vi "CALC_DATA.vi"(0 "VISA IN":refnum<visa-resource-name>="GPIB1::16::INSTR", 5 "error in":errorcluster, 7 "Channel":i32=1, 11 "DataType":string="FDATA") -> (14 "VISA Out":refnum<visa-resource-name>="GPIB1::16::INSTR", 16 "array":dbl[](array[numeric]), 19 "error out":errorcluster={"status"=TRUE, "code"=-1073807339, "source"="VISA Read in CALC_DATA.vi"})   [LabVIEW 2018, in "PNA-X.lvlib"]
doc: "CALCulate<cnum>:DATA:CUSTom <name>,<data> \n(Read-Write) Reads or writes data from a custom-named measurement buffer. \nSee Critical Note \nParameters \n<cnum> Channel number of the measurement. There must be a selected measurement \non that channel. If unspecified, <cnum> is set to 1. \n<name> Name of the buffer to be read or written \n<data> Data to be read or written to the custom buffer. Format as one number per data \npoint. \nExamples CALC:DATA:CUST 'VectorResult0',0,1,2,3,4,5 'Write \nCALC:DATA:CUST? 'VectorResult0' 'Read \nQuery Syntax CALCulate:DATA:CUSTom? <name> \nReturn Type Depends on Form:Data \nDefault Not Applicable"
uses:
  PNA-X.lvlib
panel:
  out "Waveform Chart":dbl[](graph)
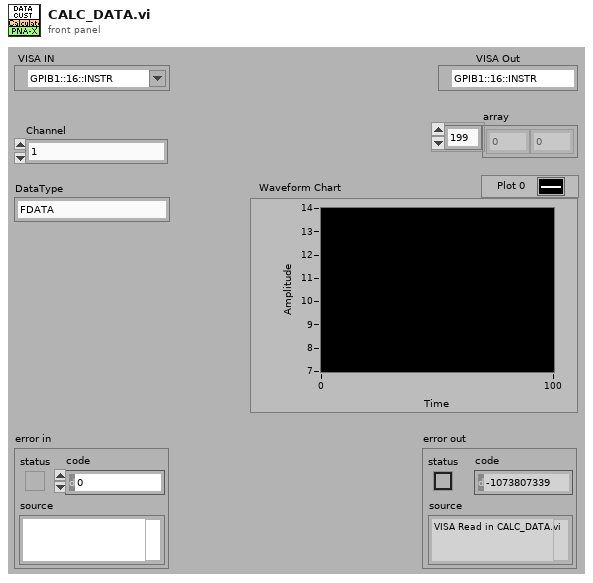
[diagram p1: front panel]
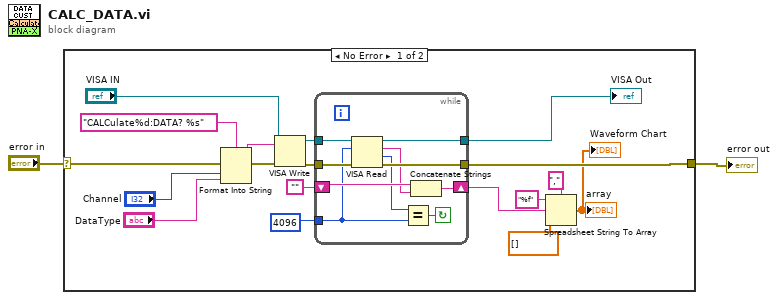
[diagram p0: block diagram]
diagram:
  n1 = case shown="No Error" "error in" {
    selector: "error in" -> [w20 w31]
    tunnel: [w11 w31] -> w1
    frame No Error {
      n2 = Format Into String(format string="CALCulate%d:DATA? %s" ("Cmdline"), error in=w20, "Channel", "DataType") -> (resulting string=w18:string, error out=w19:errorcluster)  [unwired: 1 in]
      n3 = VISA Write(VISA resource name="VISA IN", write buffer=w18, error in (no error)=w19) -> (VISA resource name out=w14:refnum<visa-resource-name>, error out=w12:errorcluster)  [unwired: 1 out]
      n4 = while {
        tunnel: w14 -> [w30]
        tunnel: [w29] -> w13
        tunnel: w12 -> [w28]
        tunnel: [w27] -> w11
        shift-right: [w25] -> w5
        shift-left: "" -> [w26]
        tunnel: u32 4096 ("byte count") -> [w22]
        stop <- w21 continue-if-true
        n5 = VISA Read(VISA resource name=w30, byte count=w22, error in (no error)=w28) -> (VISA resource name out=w29:refnum<visa-resource-name>, read buffer=w24:string, return count=w23:u32, error out=w27:errorcluster)
        n6 = Equal?(x=w23, y=w22) -> (x = y?=w21:bool)
        n7 = Concatenate Strings(w26, w24) -> (w25:string)
      }
      "VISA Out" <- w13
      n8 = Spreadsheet String To Array(delimiter (Tab)=",", format string="%f", spreadsheet string=w5, array type (2D Dbl)=dbl[] []) -> (array=→"array" →"Waveform Chart":dbl[])
    }
    frame Error {
    }
  }
  "error out" <- w1
